vi "Packet_encode_Transform3d.vi"(9 "Transform3d Value":T1={"TRANSLATION3D"={"X"=0.0, "Y"=0.0, "Z"=0.0}, "ROTATION3D"={"Q_quaternion"={"R"=1.0, "V"=[0.0, 0.0, 0.0]}}, "XF"=FALSE} {"TRANSLATION3D"."Z" format="%14.3f"; "TRANSLATION3D"."Y" format="%14.3f"; "TRANSLATION3D"."X" format="%14.3f"}, 11 "RawData In":u8[](array[numeric])) -> (3 "RawData Out":u8[](array[numeric]))   [LabVIEW 2019, in "PhotonVisionLib.lvlib"]
doc: "Encode (or append) a double floating point value (FLT 64) at the end of an array of bytes. No conversion is actually done, the memory is just copied to the end of the array.\n\nInputs\n - RawData In -- Array of bytes to be appended to..\n - FLT64_Value -- Double floating point value.\n\nOutputs\n - RawData Out -- Array of bytes containing the appended value."
uses:
  PhotonVisionLib.lvlib
  <vilib>/Rock Robotics/WPI/ThirdParty/JAS_Junk/TrajLib/TypeDef/TRANSFORM3D.ctl
  <vilib>/Rock Robotics/WPI/ThirdParty/JAS_Junk/TrajLib/TypeDef/TRANSLATION3D.ctl
  <vilib>/Rock Robotics/WPI/ThirdParty/JAS_Junk/TrajLib/TypeDef/ROTATION3D.ctl
  <vilib>/Rock Robotics/WPI/ThirdParty/JAS_Junk/TrajLib/TypeDef/QUATERNION.ctl
  <vilib>/Rock Robotics/WPI/ThirdParty/JAS_Junk/TrajLib/VI/Transform3d_GetTranslation3d.vi
  <vilib>/Rock Robotics/WPI/ThirdParty/JAS_Junk/TrajLib/VI/Translation3d_GetXYZ.vi
  <vilib>/Rock Robotics/WPI/ThirdParty/JAS_Junk/TrajLib/Trajectory_Library.lvlib
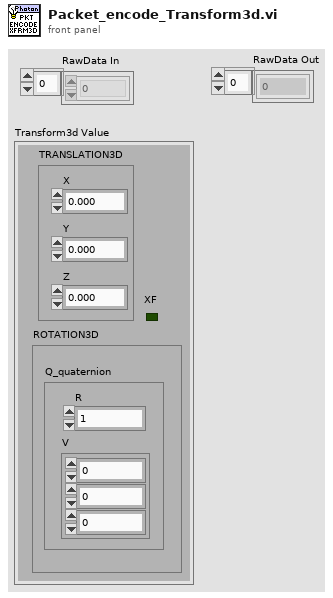
[diagram p1: front panel]
types:
  T1 = typedef "Trajectory_Library.lvlib/TRANSFORM3D.ctl" = cluster{"TRANSLATION3D":T2, "ROTATION3D":T3, "XF":bool}
  T2 = typedef "Trajectory_Library.lvlib/TRANSLATION3D.ctl" = cluster{"X":dbl, "Y":dbl, "Z":dbl}
  T3 = typedef "Trajectory_Library.lvlib/ROTATION3D.ctl" = cluster{"Q_quaternion":T4}
  T4 = typedef "Trajectory_Library.lvlib/QUATERNION.ctl" = cluster{"R":dbl, "V":dbl[]}
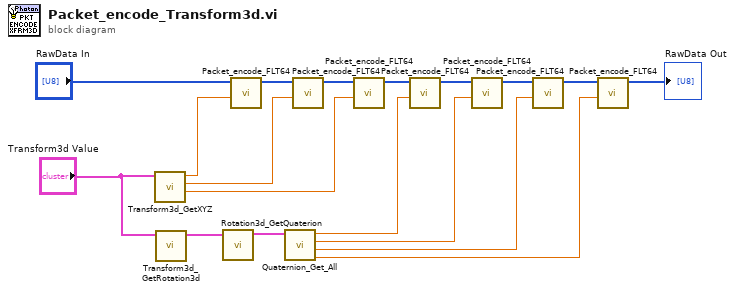
[diagram p0: block diagram]
diagram:
  n1 = call <vilib>:"Transform3d_GetXYZ.vi"("inTransform3d"="Transform3d Value") -> ("Z"=w6:dbl, "Y"=w7:dbl, "X"=w8:dbl)  [unwired: 8 in]
  n2 = call <vilib>:"Transform3d_GetRotation3d.vi"("in Transform3d"="Transform3d Value") -> ("Rotation3d"=w17:T3)  [unwired: 10 in]
  n3 = call <vilib>:"Rotation3d_GetQuaterion.vi"("in Rotation3d"=w17) -> ("out Quaterion"=w16:T4)  [unwired: 10 in]
  n4 = call "Packet_encode_FLT64.vi"("FLT64_Value"=w8, "RawData In"="RawData In") -> ("RawData Out"=w14:u8[])  [unwired: 9 in]
  n5 = call <vilib>:"Quaternion_Get_All.vi"("Quaternion"=w16) -> ("Z"=w2:dbl, "Y"=w3:dbl, "X"=w4:dbl, "W"=w5:dbl)  [unwired: 7 in]
  n6 = call "Packet_encode_FLT64.vi"("FLT64_Value"=w7, "RawData In"=w14) -> ("RawData Out"=w13:u8[])  [unwired: 9 in]
  n7 = call "Packet_encode_FLT64.vi"("FLT64_Value"=w6, "RawData In"=w13) -> ("RawData Out"=w10:u8[])  [unwired: 9 in]
  n8 = call "Packet_encode_FLT64.vi"("FLT64_Value"=w5, "RawData In"=w10) -> ("RawData Out"=w12:u8[])  [unwired: 9 in]
  n9 = call "Packet_encode_FLT64.vi"("FLT64_Value"=w4, "RawData In"=w12) -> ("RawData Out"=w11:u8[])  [unwired: 9 in]
  n10 = call "Packet_encode_FLT64.vi"("FLT64_Value"=w3, "RawData In"=w11) -> ("RawData Out"=w9:u8[])  [unwired: 9 in]
  n11 = call "Packet_encode_FLT64.vi"("FLT64_Value"=w2, "RawData In"=w9) -> ("RawData Out"=→"RawData Out":u8[])  [unwired: 9 in]
